vi "Converter_baseline_avg_to_string_indicator.vi"(8 "error in (no error)":errorcluster, 10 "Average array in":dbl[][](array[numeric]), 11 "Ref of baseline indicator":refnum<vi>) -> (0 "error out":errorcluster, 3 "Baselines per unit":T1)   [LabVIEW 2013]
uses:
  Converter_baseline_indicator.ctl
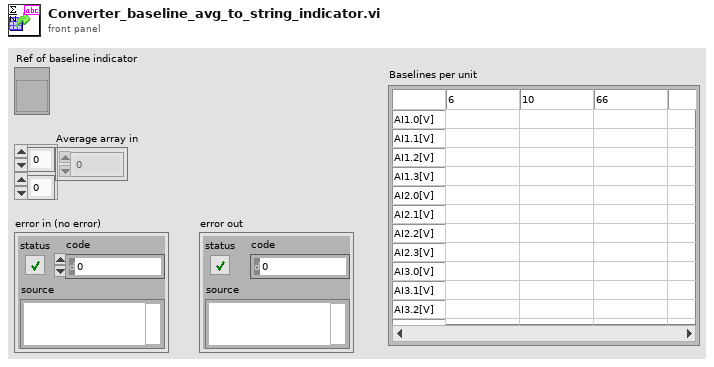
[diagram p1: front panel]
types:
  T1 = typedef "Converter_baseline_indicator.ctl" = string[][]
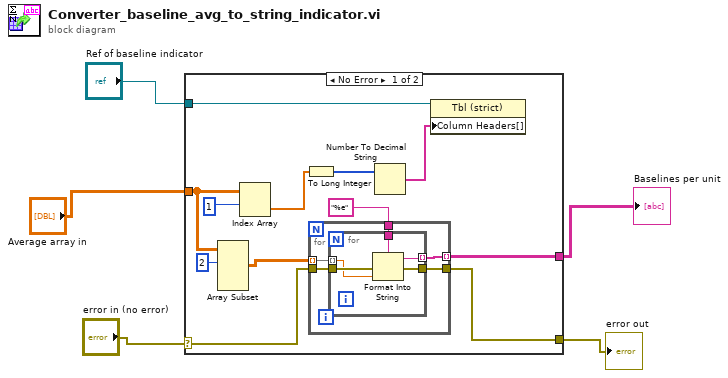
[diagram p0: block diagram]
diagram:
  n1 = case shown="No Error" "error in (no error)" {
    selector: "error in (no error)" -> [w11 w28]
    tunnel: "Average array in" -> [w12 _]
    tunnel: [w14 w28] -> w4
    tunnel: "Ref of baseline indicator" -> [w13 _]
    tunnel: [w7 _] -> w1
    frame No Error {
      n2 = Array Subset(array=w12, index (row)=2 ("index")) -> (w9:dbl[][])  [unwired: 3 in]
      n3 = Index Array(array=w12, index (row)=1) -> (element=w16:dbl[])  [unwired: 1 in]
      n4 = To Long Integer(number=w16) -> (32bit integer=w15:i32[])
      n5 = for {
        tunnel: [w22] -> w14
        tunnel: w11 -> [w21]
        tunnel: [w20] -> w7 mode=indexing
        tunnel: w9 -> [w19] mode=indexing
        tunnel: "%e" ("format string") -> [w18]
        n6 = for {
          tunnel: w21 -> [w27]
          tunnel: [w26] -> w22
          tunnel: [w25] -> w20 mode=indexing
          tunnel: w19 -> [w24] mode=indexing
          tunnel: w18 -> [w23]
          n7 = Format Into String(format string=w23, error in=w27, w24) -> (resulting string=w25:string, error out=w26:errorcluster)  [unwired: 1 in]
        }
      }
      n8 = Number To Decimal String(number=w15) -> (decimal integer string=w8:string[])  [unwired: 1 in]
      n9 = property class="Tbl (strict)"(reference=w13, "Column Headers[]"=w8) -> ()  [unwired: 1 in, 2 out]
    }
    frame Error {
    }
  }
  "error out" <- w4
  "Baselines per unit" <- w1
